vi "Write sub-VI.vi"(7 "Port to Write (RT)":enum8{"1", "2", "3", "4"}(ring) caption="Port", 8 "Write sub-VI Error In":errorcluster, 9 "Write Data?":bool, 10 "String To Write":string, 11 "FPGA VI Reference In":refnum<k20>) -> (0 "Write sub-VI Error Out":errorcluster, 3 "FPGA VI Reference Out":refnum<k20>)   [LabVIEW 2012]
doc: "Writes the data from the \"String To Write\" String Control to the WRITE_FIFO hosted on the FPGA when the \"Write Data\" button is pressed."
uses:
  <vilib>/Utility/error.llb/Error Cluster From Error Code.vi
  <vilib>/rvi/errors/niLvFpgaAdjustHostInterfaceError.vi
  <vilib>/rvi/interface/nirviReadWriteControl/nirviReadWriteControl.xnode
  <vilib>/rvi/interface/nirviMethod/nirviMethod.xnode
  NiFpgaLv.dll
  <vilib>/rvi/interface/Simulation/niFpgaSimulationCallBeginRW.vi
  <vilib>/FPGAPlugInAG/Dynamic/niLvFpga_WriteFifo_Dynamic.vi
  <vilib>/rvi/errors/niLvFpgaMergeErrorWithErrorCode.vi
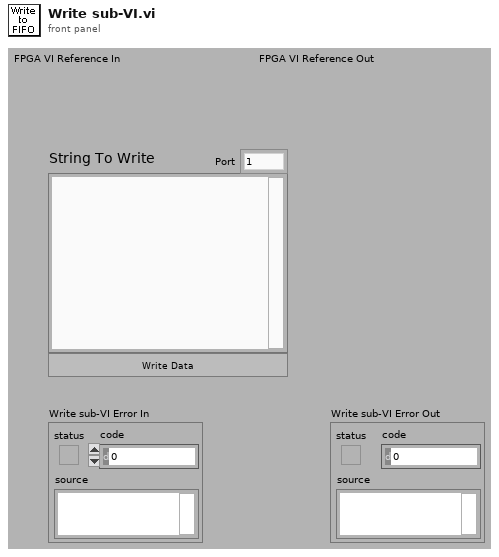
[diagram p1: front panel]
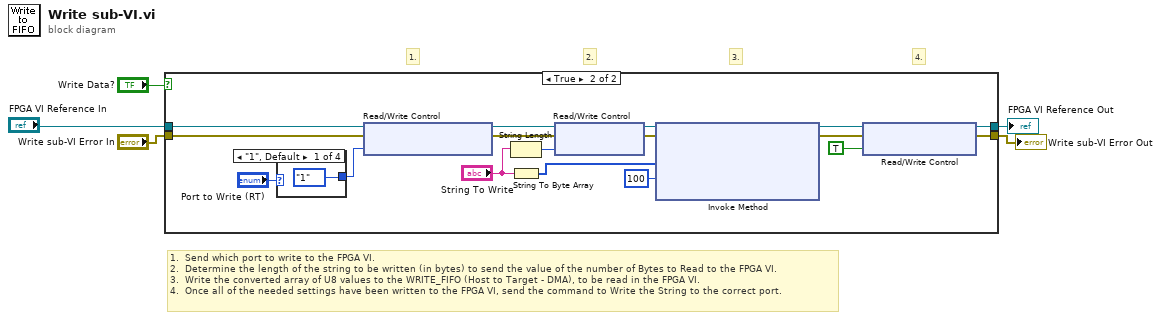
[diagram p0: block diagram]
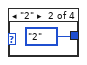
[diagram p3: hidden frame]
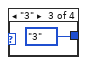
[diagram p4: hidden frame]
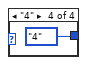
[diagram p5: hidden frame]
diagram:
  # "1.  Send which port to write to the FPGA VI.\n2.  Determine the length of the string to be written (in bytes) to send the value of the number of Bytes to Read to the FPGA VI.\n3.  Write the converted array of U8 values to the WRITE_FIFO (Host to Target - DMA), to be read in the FPGA VI.\n4.  Once all of the needed settings have been written to the FPGA VI, send the command to Write the String to the correct port."
  # "4."
  # "3."
  # "2."
  # "1."
  n1 = case shown="True" "Write Data?" {
    tunnel: "FPGA VI Reference In" -> [w7 w14]
    tunnel: [w7 w17] -> w1
    tunnel: "Write sub-VI Error In" -> [w6 w13]
    tunnel: [w6 w18] -> w3
    frame False {
    }
    frame True {
      n2 = case shown="\"1\", Default" "Port to Write (RT)" {
        tunnel: [enum8{"0", "1", "2", "3", "4"}."1" ("Port To Write (FPGA)") enum8{"0", "1", "2", "3", "4"}."2" ("Port To Write (FPGA)") enum8{"0", "1", "2", "3", "4"}."3" ("Port To Write (FPGA)") enum8{"0", "1", "2", "3", "4"}."4" ("Port To Write (FPGA)")] -> w8
        frame "1", Default {
        }
        frame "2" {
        }
        frame "3" {
        }
        frame "4" {
        }
      }
      n3 = xnode "Read/Write Control"("FPGA VI Reference In"=w14, "error in"=w13, "Port To Write (FPGA)"=w8) -> ("FPGA VI Reference Out"=w15:refnum<k20>, "error out"=w16:errorcluster)
      n4 = String Length(string="String To Write") -> (length=w21:i32)
      n5 = String To Byte Array(string="String To Write") -> (unsigned byte array=w23:u8[])
      n6 = xnode "Read/Write Control"("FPGA VI Reference In"=w15, "error in"=w16, "Bytes to Send"=w21) -> ("FPGA VI Reference Out"=w11:refnum<k20>, "error out"=w12:errorcluster)
      n7 = xnode "Invoke Method"("FPGA VI Reference In"=w11, "error in"=w12, "Data"=w23, "Timeout (ms)"=100) -> ("FPGA VI Reference Out"=w20:refnum<k20>, "error out"=w19:errorcluster)  [unwired: 1 out]
      n8 = xnode "Read/Write Control"("FPGA VI Reference In"=w20, "error in"=w19, "Write Data (FPGA)"=TRUE) -> ("FPGA VI Reference Out"=w17:refnum<k20>, "error out"=w18:errorcluster)
    }
  }
  "Write sub-VI Error Out" <- w3
  "FPGA VI Reference Out" <- w1
